vi "LINX_servo.vi"(9 "Servo Channel":u8=9, 10 "Serial Port":refnum<visa-resource-name>="COM4", 11 "Boolean":bool) -> (3 "Shatter Open":bool)   [LabVIEW 2015]
doc: "This example demonstrates how to control a servo using LINX."
uses:
  <vilib>/MakerHub/LINX/Public/Utilities/Open Serial.vi
  <vilib>/MakerHub/LINX/Public/Sensors/Motion/Servo/Servo Open One Channel.vi
  <vilib>/MakerHub/LINX/Public/Sensors/Motion/Servo/Servo Set Pulse Width One Channel.vi
  <vilib>/MakerHub/LINX/Public/Sensors/Motion/Servo/Servo Close One Channel.vi
  <vilib>/MakerHub/LINX/LMH-LINX.lvlib
  <vilib>/MakerHub/LINX/Public/Sensors/Motion/Servo/Servo.lvlib
  <vilib>/Analysis/NI_AALPro.lvlib
panel:
  in  "Servo Position":u16(knob)=1493 scale=500.0..2500.0
  in  "Stop Button 2":bool
  # "Servo Example (Serial Interface)\n\nThis example demonstrates how to control a servo.\n\nInstructions\n1. Select the COM Port associated with the LINX Device.\n2. Select the Servo Channel connected to the servo to control.\n3. Click the Run Arrow.\n4. Adjust the dial to control the digital pulse width sent to the servo.  The pulse \n    width determines the servo position.  A 1500 uS pulse is typically 90 degrees.  \n    The maximum angle will depend on the sepcific servo used."
  # "Servo Position \n(Pulse Width uS)"
  # "LINX Device Settings"
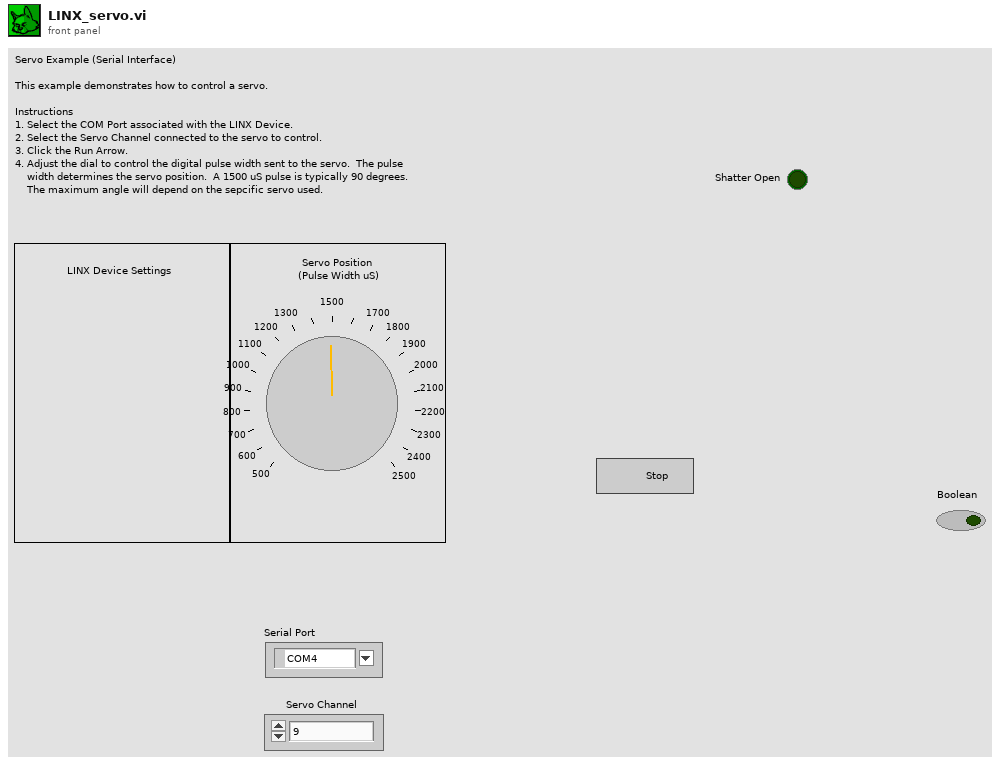
[diagram p1: front panel]
types:
  T1 = typedef "LMH-LINX.lvlib/LINX Ref.ctl" = cluster{"IO":T2, "Interface":T3, "LINX Device Config":T4}
  T2 = typedef "LMH-LINX.lvlib/Platform.ctl" = enum16{"Remote", "Local"}
  T3 = typedef "LMH-LINX.lvlib/Interface.ctl" = enum16{"Serial", "TCP"}
  T4 = typedef "LMH-LINX.lvlib/Device.lvlib/LINX Device Config.ctl" = cluster{"Interface":T3, "COM Port":refnum<visa-resource-name>, "TCP Configuration":T5, "Device Family":u8, "Device ID":u8, "Device Name":string, "TCP Ref":refnum<k5>, "Channels":T6}
  T5 = typedef "LMH-LINX.lvlib/Device.lvlib/TCP Config.ctl" = cluster{"IP Address":string, "Port":u16}
  T6 = typedef "LMH-LINX.lvlib/Channels.ctl" = cluster{"DI":u8[], "DO":u8[], "AI":u8[], "AO":u8[], "PWM":u8[], "QE":u8[], "UART":u8[], "I2C 2":u8[], "SPI":u8[], "CAN":u8[], "Servo":u8[], "AI Ref (V)":dbl, "AI Resolution (Bits)":u8, "AO Ref (V)":dbl, "AO Resolution (Bits)":u8}
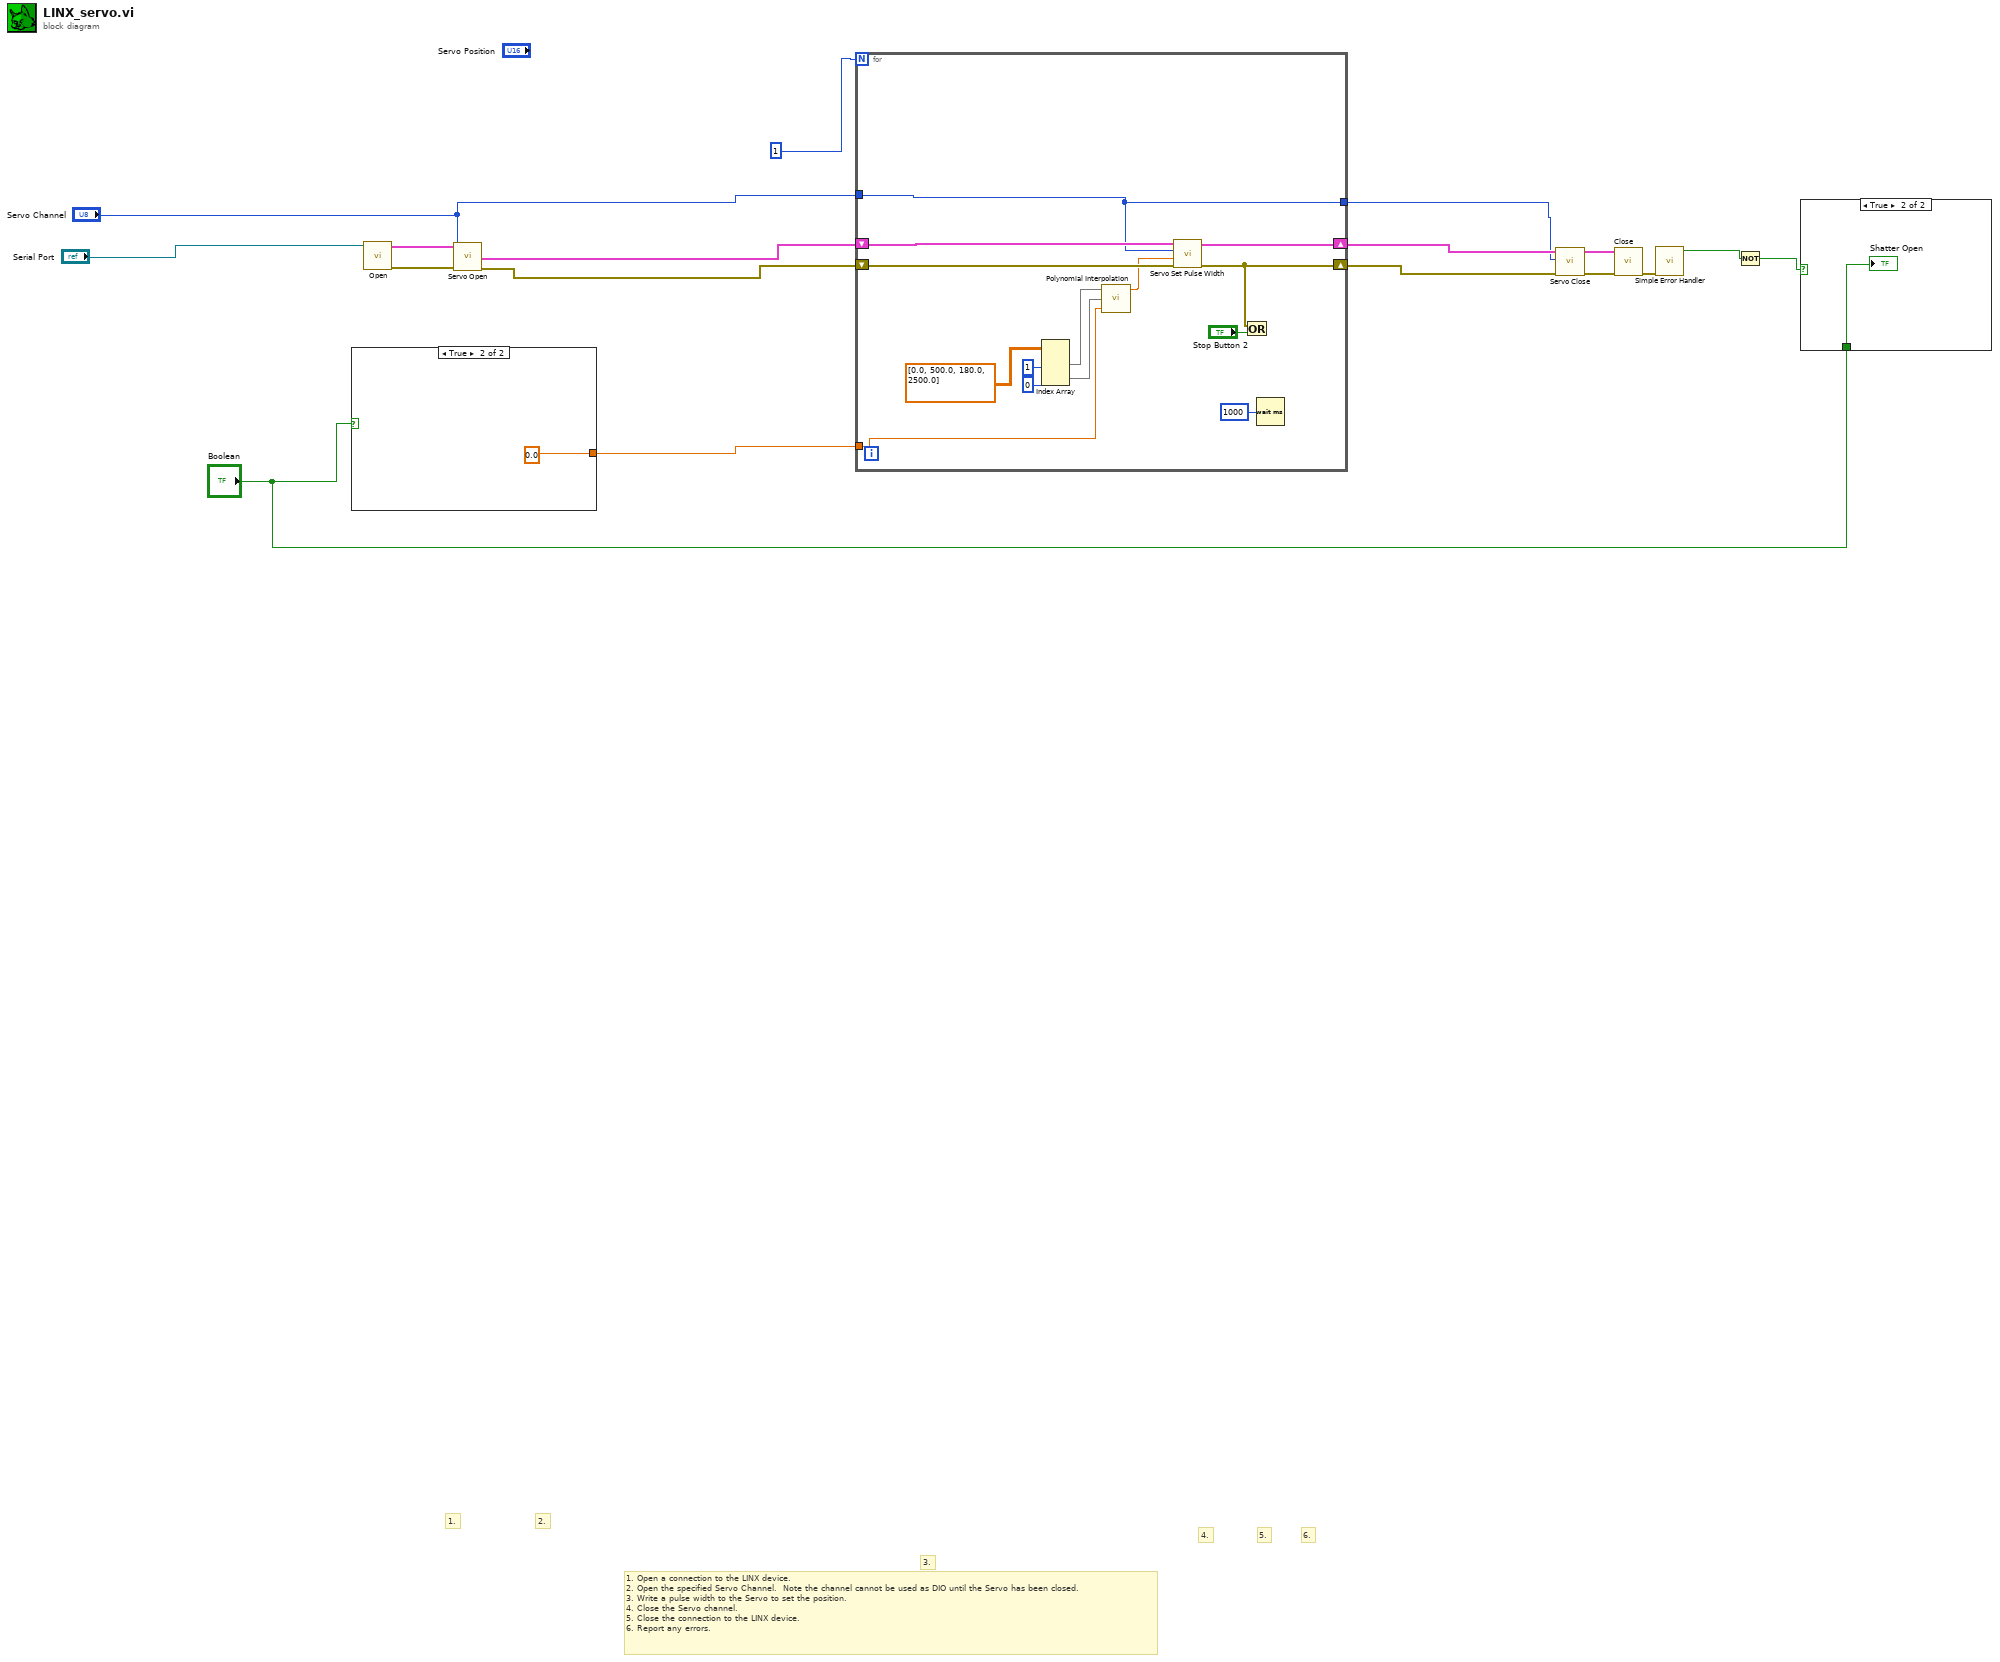
[diagram p0: block diagram]
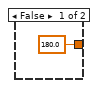
[diagram p3: hidden frame]
diagram:
  # "6."
  # "1. Open a connection to the LINX device.\n2. Open the specified Servo Channel.  Note the channel cannot be used as DIO until the Servo has been closed.\n3. Write a pulse width to the Servo to set the position.\n4. Close the Servo channel.  \n5. Close the connection to the LINX device.\n6. Report any errors."
  # "5."
  # "4."
  # "3."
  # "2."
  # "1."
  n1 = case shown="True" "Boolean" {
    tunnel: [180.0 ("x value") 0.0 ("x value")] -> w14
    frame False {
    }
    frame True {
    }
  }
  n2 = call-poly <vilib>:"Open.vi"("Serial Port"="Serial Port") -> ("Error Out"=w13:errorcluster, "LINX Resource"=w12:T1)  [unwired: 8 in, 1 out]
  n3 = call-poly <vilib>:"Servo Open.vi"("Error In"=w13, "Servo Channel"="Servo Channel", "LINX Resource"=w12) -> ("Error Out"=w15:errorcluster, "LINX Resource"=w16:T1)  [unwired: 7 in]
  n4 = for {
    N: 1 -> [_]
    tunnel: "Servo Channel" -> [w23]
    tunnel: w14 -> [w21]
    shift-right: [w33] -> w9
    shift-left: w16 -> [w25]
    shift-right: [w32] -> w6
    shift-left: w15 -> [w24]
    tunnel: [w23] -> w5
    n5 = Index Array(array=dbl[][] [[0.0, 500.0], [180.0, 2500.0]], index (col) #1=1 ("disabled index (col)"), index (col) #2=0 ("index (col)")) -> (element #1=w29:dbl[], element #2=w28:dbl[])  [unwired: 2 in]
    n6 = call <vilib>:"Polynomial Interpolation.vi"("x value"=w21, "X"=w28, "Y"=w29) -> ("interpolation value"=w20:dbl)  [unwired: 2 out]
    n7 = call-poly <vilib>:"Servo Set Pulse Width.vi"("Error In"=w24, "Pulse Width (uS)"=w20, "Servo Channel"=w23, "LINX Resource"=w25) -> ("Error Out"=w32:errorcluster, "LINX Resource"=w33:T1)  [unwired: 6 in]
    n8 = Or(x=w32, y="Stop Button 2") -> ()  [unwired: 1 out]
    n9 = Wait (ms)(milliseconds to wait=u32 1000) -> ()  [unwired: 1 out]
  }
  n10 = call-poly <vilib>:"Servo Close.vi"("Error In"=w6, "Servo Channel"=w5, "LINX Resource"=w9) -> ("Error Out"=w7:errorcluster, "LINX Resource"=w8:T1)  [unwired: 7 in]
  n11 = call <vilib>:"Close.vi"("Error In"=w7, "LINX Resource"=w8) -> ("Error Out"=w10:errorcluster)  [unwired: 9 in]
  n12 = call <vilib>:"Simple Error Handler.vi"("error in (no error)"=w10) -> ("error?"=w4:bool)  [unwired: 4 in, 4 out]
  n13 = Not(x=w4) -> (.not. x?=w3:bool)
  n14 = case shown="True" w3 {
    tunnel: "Boolean" -> [_ w34]
    frame False {
    }
    frame True {
      "Shatter Open" <- w34
    }
  }
